vi "Convert_sequence_line_to_command.vi"(8 "Sample Handler Configuration":T3={"port"="", "BG 1"=82130, "BG 2"=22570, "Sensor"=74765, "AF 1"=51160, "AF 2"=123198, "AF coil"=110030, "Home (absolute)"=72, "Home (relative to limit switch)"=990, "robot"=40750}, 9 "Current status":T1, 10 "Sample offset":u16[](array[numeric]), 11 "sequence line":string) -> (3 "コマンド配列":string[](array[string]))   [LabVIEW 2017]
uses:
  controls/SampleHandler_configuration.ctl
  controls/Curret_status.ctl
  controls/wait_mode.ctl
panel:
  in  "ダミー":string[](array[string])
  # "Count (Positive=RH)"
  # "Relative to Home?"
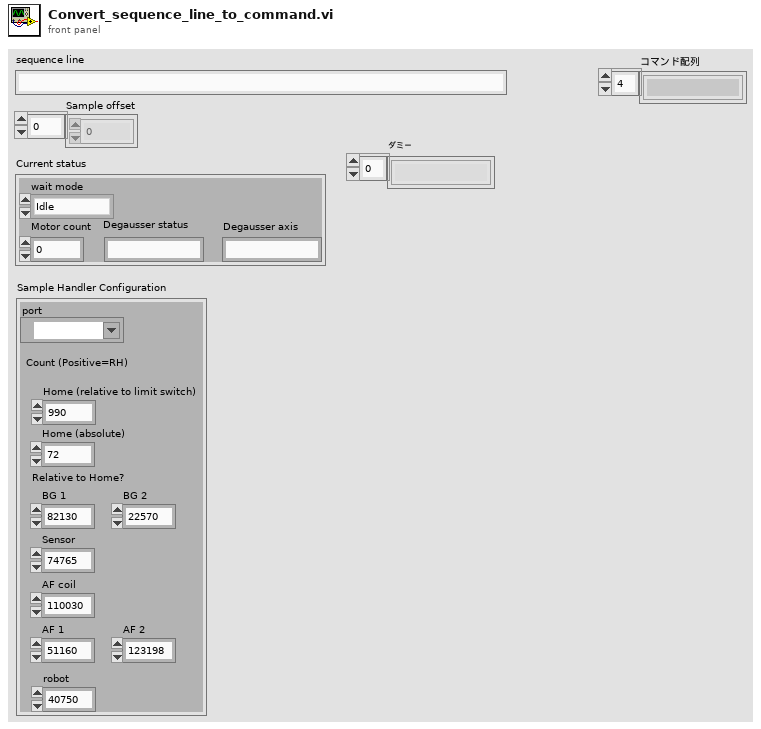
[diagram p1: front panel]
types:
  T1 = typedef "Curret_status.ctl" = cluster{"Motor count":i32, "Degausser status":string, "Degausser axis":string, "wait mode":T2}
  T2 = typedef "wait_mode.ctl" = enum16{"Idle", "Executing", "Moving", "Homing", "Zeroing", "Ramping", "Robot", "Pause"}
  T3 = typedef "SampleHandler_configuration.ctl" = cluster{"port":refnum<visa-resource-name>, "BG 1":i32, "BG 2":i32, "Sensor":i32, "AF 1":i32, "AF 2":i32, "AF coil":i32, "Home (absolute)":i32, "Home (relative to limit switch)":i32, "robot":i32}
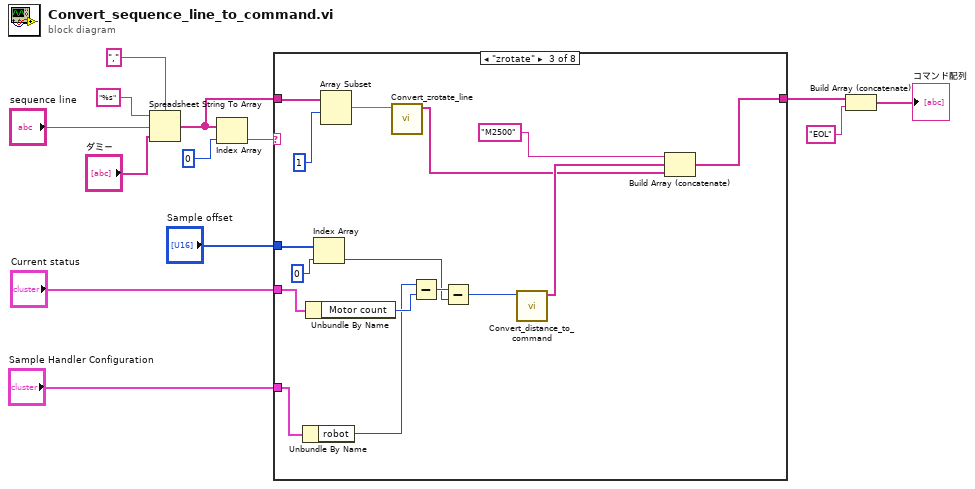
[diagram p0: block diagram]
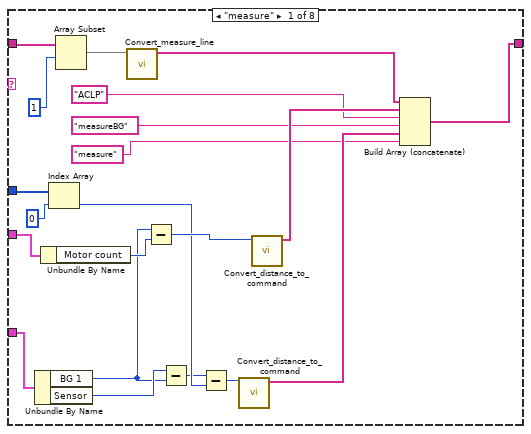
[diagram p2: hidden frame]
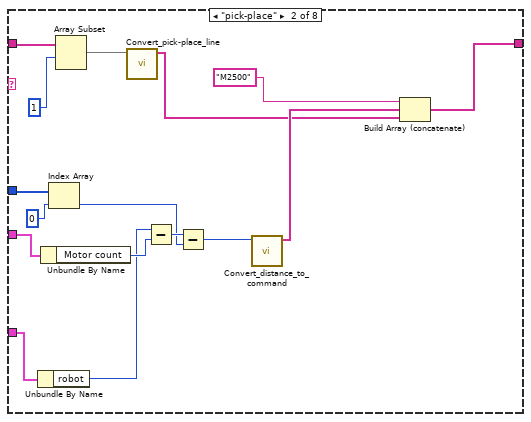
[diagram p3: hidden frame]
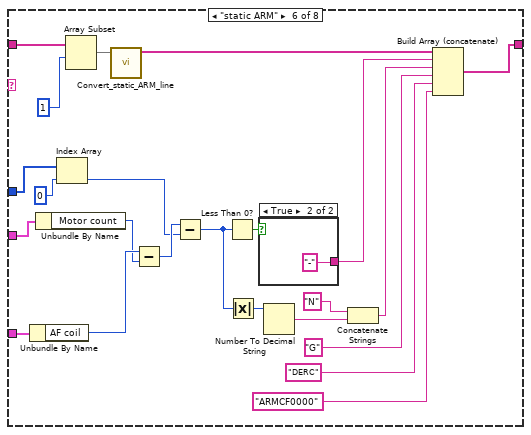
[diagram p6: hidden frame]
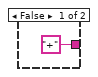
[diagram p7: hidden frame]
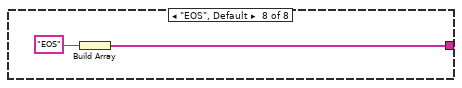
[diagram p9: hidden frame]
diagram:
  n1 = Spreadsheet String To Array(delimiter (Tab)=",", format string="%s", spreadsheet string="sequence line", array type (2D Dbl)="ダミー") -> (array=w8:string[])
  n2 = Index Array(array=w8, index=0) -> (element=w7:string)
  n3 = case shown="\"zrotate\"" w7 {
    tunnel: w8 -> [w21 w39 w55 w67 w68 w90 w94 _]
    tunnel: [w18 w46 w62 w67 w68 w69 w94 w95] -> w6
    tunnel: "Sample Handler Configuration" -> [w32 w48 w64 _ _ w83 _ _]
    tunnel: "Current status" -> [w33 w49 w65 _ _ w82 _ _]
    tunnel: "Sample offset" -> [w30 w44 w60 _ _ w73 _ _]
    frame "measure" {
      n4 = Unbundle By Name(w32) -> ("BG 1"=w28:i32, "Sensor"=w29:i32)
      n5 = Unbundle By Name(w33) -> ("Motor count"=w34:i32)
      n6 = Index Array(array=w30, index=0) -> (element=w15:u16)
      n7 = Array Subset(array=w21, index=1) -> (w20:string[])  [unwired: 1 in]
      n8 = call "Convert_measure_line.vi"("sequence line"=w20) -> ("command"=w19:string[])  [unwired: 10 in]
      n9 = Subtract(x=w28, y=w34) -> (x-y=w17:i32)
      n10 = Subtract(x=w29, y=w28) -> (x-y=w14:i32)
      n11 = Subtract(x=w14, y=w15) -> (x-y=w16:i32)
      n12 = call "Convert_distance_to_command.vi"("relative count"=w16) -> ("command"=w26:string[])  [unwired: 10 in]
      n13 = call "Convert_distance_to_command.vi"("relative count"=w17) -> ("command"=w27:string[])  [unwired: 10 in]
      n14 = Build Array (concatenate)(w19, w27, "ACLP", "measureBG", w26, "measure") -> (w18:string[])
    }
    frame "pick-place" {
      n15 = Unbundle By Name(w48) -> ("robot"=w38:i32)
      n16 = Unbundle By Name(w49) -> ("Motor count"=w50:i32)
      n17 = Index Array(array=w44, index=0) -> (element=w43:u16)
      n18 = Array Subset(array=w39, index=1) -> (w36:string[])  [unwired: 1 in]
      n19 = call "Convert_pick-place_line.vi"("sequence line"=w36) -> ("command"=w35:string[])  [unwired: 10 in]
      n20 = Subtract(x=w38, y=w50) -> (x-y=w47:i32)
      n21 = Subtract(x=w47, y=w43) -> (x-y=w42:i32)
      n22 = call "Convert_distance_to_command.vi"("relative count"=w42) -> ("command"=w41:string[])  [unwired: 10 in]
      n23 = Build Array (concatenate)("M2500", w41, w35) -> (w46:string[])
    }
    frame "zrotate" {
      n24 = Unbundle By Name(w64) -> ("robot"=w54:i32)
      n25 = Unbundle By Name(w65) -> ("Motor count"=w66:i32)
      n26 = Index Array(array=w60, index=0) -> (element=w59:u16)
      n27 = Array Subset(array=w55, index=1) -> (w52:string[])  [unwired: 1 in]
      n28 = call "Convert_zrotate_line.vi"("sequence line"=w52) -> ("command"=w51:string[])  [unwired: 10 in]
      n29 = Subtract(x=w54, y=w66) -> (x-y=w63:i32)
      n30 = Subtract(x=w63, y=w59) -> (x-y=w58:i32)
      n31 = call "Convert_distance_to_command.vi"("relative count"=w58) -> ("command"=w57:string[])  [unwired: 10 in]
      n32 = Build Array (concatenate)("M2500", w57, w51) -> (w62:string[])
    }
    frame "static AFD" {
    }
    frame "pass through AFD" {
    }
    frame "static ARM" {
      n33 = Unbundle By Name(w83) -> ("AF coil"=w85:i32)
      n34 = Unbundle By Name(w82) -> ("Motor count"=w76:i32)
      n35 = Index Array(array=w73, index=0) -> (element=w71:u16)
      n36 = Array Subset(array=w90, index=1) -> (w89:string[])  [unwired: 1 in]
      n37 = call "Convert_static_ARM_line.vi"("sequence line"=w89) -> ("コマンド配列"=w81:string[])  [unwired: 9 in]
      n38 = Subtract(x=w85, y=w76) -> (x-y=w75:i32)
      n39 = Subtract(x=w75, y=w71) -> (x-y=w74:i32)
      n40 = Less Than 0?(x=w74) -> (x < 0?=w86:bool)
      n41 = Absolute Value(x=w74) -> (abs(x)=w87:i32)
      n42 = case shown="TRUE" w86 {
        tunnel: ["+" "-"] -> w80
        frame False {
        }
        frame True {
        }
      }
      n43 = Number To Decimal String(number=w87) -> (decimal integer string=w88:string)  [unwired: 1 in]
      n44 = Concatenate Strings("N", w88) -> (w79:string)
      n45 = Build Array (concatenate)(w81, w80, w79, "G", "DERC", "ARMCF0000") -> (w69:string[])
    }
    frame "pass through ARM" {
    }
    frame "EOS", Default {
      n46 = Build Array("EOS") -> (w95:string[])
    }
  }
  n47 = Build Array (concatenate)(w6, "EOL") -> (→"コマンド配列":string[])
